vi "Build-timeline.vi"(8 "error in (no error)":errorcluster, 10 "Temp-timeline in":T1={"Previous point"={"Start time [µs]"=0, "End time [µs]"=0, "X [mm]"=0.0, "Y [mm]"=0.0, "Type"=enum."BeginJob", "Speed [mm/µs]"=0.0, "Direction [rad]"=0.0, "X [bit]"=0, "Y [bit]"=0, "Speed [bit/µs]"=0.0, "Power [W]"=0.0, "Power [bit]"=0, "JumpDelay"=0, "MarkDelay"=0, "PolyDelay"=0, "LaserOnDelay"=0, "LaserOffDelay"=0, "LaserPowerDelay"=0, "LaserEnableDelay"=0, "Xraw [mm]"=0.0, "Yraw [mm]"=0.0}, "Current point"={"Start time [µs]"=0, "End time [µs]"=0, "X [mm]"=0.0, "Y [mm]"=0.0, "Type"=enum."BeginJob", "Speed [mm/µs]"=0.0, "Direction [rad]"=0.0, "X [bit]"=0, "Y [bit]"=0, "Speed [bit/µs]"=0.0, "Power [W]"=0.0, "Power [bit]"=0, "JumpDelay"=0, "MarkDelay"=0, "PolyDelay"=0, "LaserOnDelay"=0, "LaserOffDelay"=0, "LaserPowerDelay"=0, "LaserEnableDelay"=0, "Xraw [mm]"=0.0, "Yraw [mm]"=0.0}, "Path"=[], "Current properties"={"ItemID"=0, "Start time"=0, "EffectiveOffset"=[0.0, 0.0], "EffectiveTranfsorm"=[[1.0, 0.0], [0.0, 1.0]], "Z-Offset"=0.0, "Units"=enum."mm", "LaserPower"=0, "Started"=FALSE, "Enabled"=FALSE, "FieldOffset"=[0.0, 0.0], "Offset"=[0.0, 0.0], "TransformEnable"=TRUE, "XYCalFactor"=196.0, "JumpSpeed"={"unit/us"=0.0, "Tick interval us"=0, "Bits per interval"=0}, "MarkSpeed"={"unit/us"=0.0, "Tick interval us"=0, "Bits per interval"=0}}}, 11 "JumpAbs in":refnum<class "JumpRel.lvclass">) -> (0 "error out":errorcluster, 2 "Temp-timeline":T1={"Previous point"={"Start time [µs]"=0, "End time [µs]"=0, "X [mm]"=0.0, "Y [mm]"=0.0, "Type"=enum."BeginJob", "Speed [mm/µs]"=0.0, "Direction [rad]"=0.0, "X [bit]"=0, "Y [bit]"=0, "Speed [bit/µs]"=0.0, "Power [W]"=0.0, "Power [bit]"=0, "JumpDelay"=0, "MarkDelay"=0, "PolyDelay"=0, "LaserOnDelay"=0, "LaserOffDelay"=0, "LaserPowerDelay"=0, "LaserEnableDelay"=0, "Xraw [mm]"=0.0, "Yraw [mm]"=0.0}, "Current point"={"Start time [µs]"=0, "End time [µs]"=0, "X [mm]"=0.0, "Y [mm]"=0.0, "Type"=enum."BeginJob", "Speed [mm/µs]"=0.0, "Direction [rad]"=0.0, "X [bit]"=0, "Y [bit]"=0, "Speed [bit/µs]"=0.0, "Power [W]"=0.0, "Power [bit]"=0, "JumpDelay"=0, "MarkDelay"=0, "PolyDelay"=0, "LaserOnDelay"=0, "LaserOffDelay"=0, "LaserPowerDelay"=0, "LaserEnableDelay"=0, "Xraw [mm]"=0.0, "Yraw [mm]"=0.0}, "Path"=[], "Current properties"={"ItemID"=0, "Start time"=0, "EffectiveOffset"=[0.0, 0.0], "EffectiveTranfsorm"=[[1.0, 0.0], [0.0, 1.0]], "Z-Offset"=0.0, "Units"=enum."mm", "LaserPower"=0, "Started"=FALSE, "Enabled"=FALSE, "FieldOffset"=[0.0, 0.0], "Offset"=[0.0, 0.0], "TransformEnable"=TRUE, "XYCalFactor"=196.0, "JumpSpeed"={"unit/us"=0.0, "Tick interval us"=0, "Bits per interval"=0}, "MarkSpeed"={"unit/us"=0.0, "Tick interval us"=0, "Bits per interval"=0}}}, 3 "JumpAbs out":refnum<class "JumpRel.lvclass">)   [LabVIEW 2013, in "MaterialCharacterization.lvlib" / "JumpRel.lvclass"]
uses:
  JumpRel.lvclass
  ScanParser/Path-buffer.ctl
  ScanParser/Point-buffer.ctl
  Elements.ctl
  ScanParser/Property-buffer.ctl
  ScanParser/Units.ctl
  ScanParser/Speed.ctl
  JumpRel.lvclass/JumpRel.ctl
  <vilib>/Analysis/baseanly.llb/A x Vector.vi
  <vilib>/Analysis/Matrix/Numeric/Conversions/Array To Matrix - RA2.vi
  <vilib>/Analysis/Matrix/NI_Matrix.lvlib
  <vilib>/Analysis/NI_AALBase.lvlib
  Element-XML.lvclass
  ScanParser/MC-ScanParser.lvclass
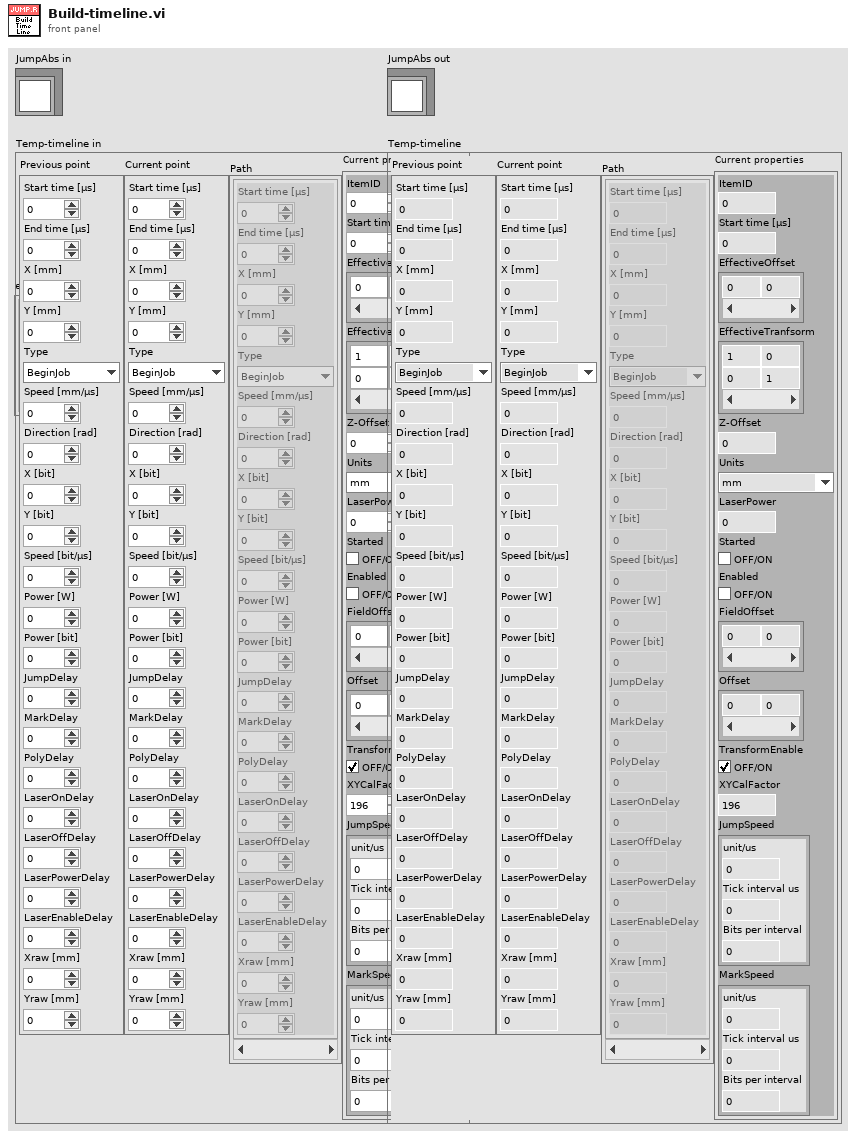
[diagram p1: front panel]
types:
  T1 = typedef "MaterialCharacterization.lvlib/MC-ScanParser.lvclass/Path-buffer.ctl" = cluster{"Previous point":T2, "Current point":T2, "Path":T2[], "Current properties":T4}
  T2 = typedef "MaterialCharacterization.lvlib/MC-ScanParser.lvclass/Point-buffer.ctl" = cluster{"Start time [µs]":i64, "End time [µs]":i64, "X [mm]":dbl, "Y [mm]":dbl, "Type":T3, "Speed [mm/µs]":dbl, "Direction [rad]":dbl, "X [bit]":i16, "Y [bit]":i16, "Speed [bit/µs]":dbl, "Power [W]":dbl, "Power [bit]":u8, "JumpDelay":i64, "MarkDelay":i64, "PolyDelay":i64, "LaserOnDelay":i64, "LaserOffDelay":i64, "LaserPowerDelay":i64, "LaserEnableDelay":i64, "Xraw [mm]":dbl, "Yraw [mm]":dbl}
  T3 = typedef "MaterialCharacterization.lvlib/Element-XML.lvclass/Elements.ctl" = enum16{"BeginJob", "WriteDigital", "WriteAnalog", "Set", "ApplicationEvent", "JumpAbs", "MarkAbs", "JumpRel", "MarkRel", "LongDelay", "EndJob"}
  T4 = typedef "MaterialCharacterization.lvlib/MC-ScanParser.lvclass/Property-buffer.ctl" = cluster{"ItemID":u32, "Start time":i64, "EffectiveOffset":dbl[], "EffectiveTranfsorm":dbl[][], "Z-Offset":sgl, "Units":T5, "LaserPower":u8, "Started":bool, "Enabled":bool, "FieldOffset":dbl[], "Offset":dbl[], "TransformEnable":bool, "XYCalFactor":dbl, "JumpSpeed":T6, "MarkSpeed":T6}
  T5 = typedef "MaterialCharacterization.lvlib/MC-ScanParser.lvclass/Units.ctl" = enum16{"bits", "mm", "inch", "mils"}
  T6 = typedef "MaterialCharacterization.lvlib/MC-ScanParser.lvclass/Speed.ctl" = cluster{"unit/us":dbl, "Tick interval us":u16, "Bits per interval":u16}
  T7 = typedef "NI_Matrix.lvlib/RealMatrix.ctl" = dbl[][]
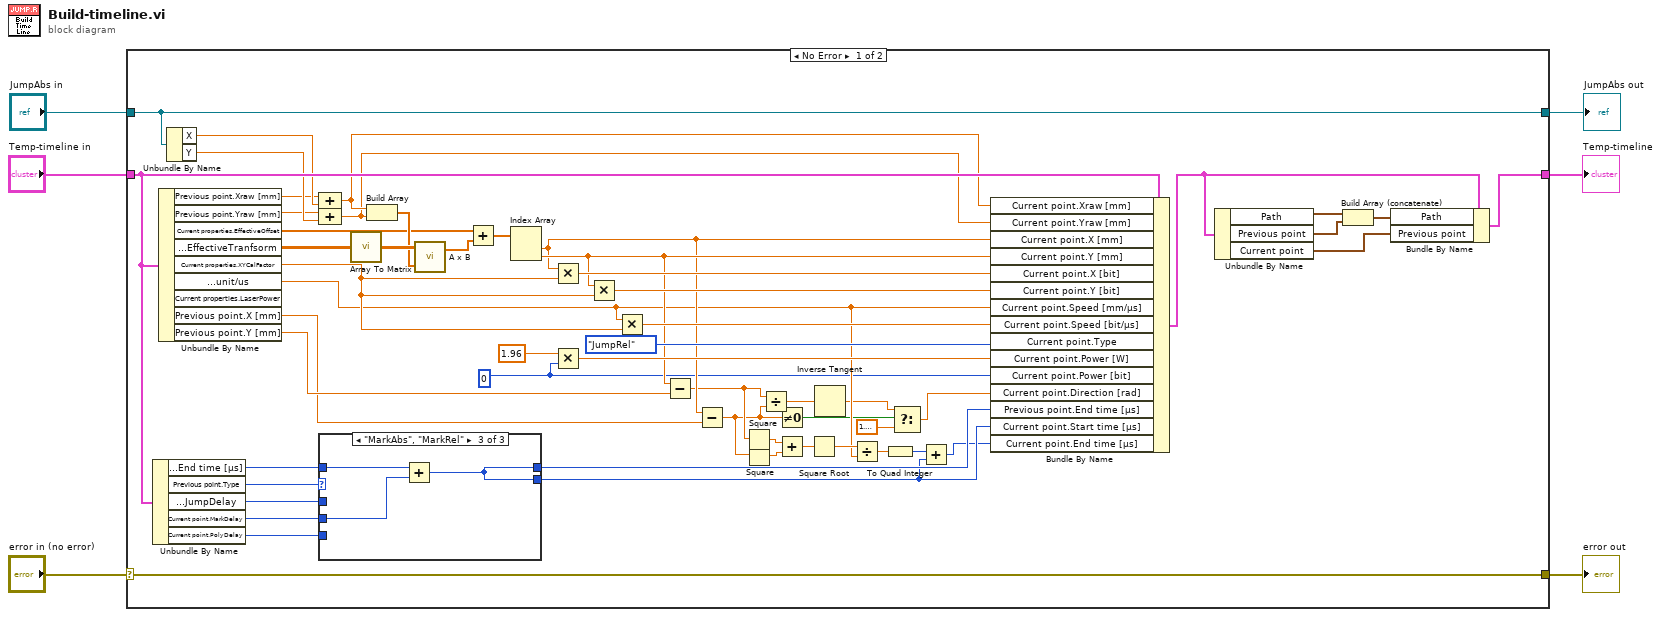
[diagram p0: block diagram]
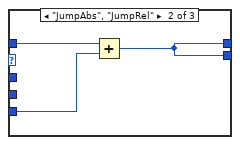
[diagram p3: hidden frame]
diagram:
  n1 = case shown="No Error" "error in (no error)" {
    selector: "error in (no error)" -> [w25 w71]
    tunnel: [w25 w71] -> w5
    tunnel: [w61 w70] -> w3
    tunnel: "JumpAbs in" -> [w61 w70]
    tunnel: "Temp-timeline in" -> [w42 w69]
    tunnel: [w23 w69] -> w1
    frame No Error {
      w18 = u8 0
      n2 = Unbundle By Name(w42) -> ("Previous point.End time [µs]"=w37:i64, "Previous point.Type"=w41:T3, "Current point.JumpDelay"=w40:i64, "Current point.MarkDelay"=w39:i64, "Current point.PolyDelay"=w38:i64)
      n3 = Unbundle By Name(w42) -> ("Previous point.Xraw [mm]"=w15:dbl, "Previous point.Yraw [mm]"=w14:dbl, "Current properties.EffectiveOffset"=w57:dbl[], "Current properties.EffectiveTranfsorm"=w60:dbl[][], "Current properties.XYCalFactor"=w51:dbl, "Current properties.JumpSpeed.unit/us"=w30:dbl, "Previous point.X [mm]"=w44:dbl, "Previous point.Y [mm]"=w46:dbl)  [unwired: 1 out]
      n4 = Unbundle By Name(w61) -> ("X"=w16:dbl, "Y"=w17:dbl)
      n5 = Compound Arithmetic op=ADD(w15, w16) -> (w13:dbl)
      n6 = Compound Arithmetic op=ADD(w14, w17) -> (w12:dbl)
      n7 = case shown="\"MarkAbs\", \"MarkRel\"" w41 {
        tunnel: w40 -> [_ _ _]
        tunnel: w39 -> [_ _ w66]
        tunnel: w38 -> [_ w64 _]
        tunnel: w37 -> [w62 w65 w68]
        tunnel: [w62 w63 w67] -> w36
        tunnel: [w62 w63 w67] -> w27
        frame "BeginJob", Default {
        }
        frame "JumpAbs", "JumpRel" {
          n8 = Add(x=w65, y=w64) -> (x+y=w63:i64)
        }
        frame "MarkAbs", "MarkRel" {
          n9 = Add(x=w68, y=w66) -> (x+y=w67:i64)
        }
      }
      n10 = call-poly <vilib>:"Array To Matrix.vi"("Real 2D Array"=w60) -> ("Real Matrix"=w59:T7)
      n11 = Build Array(w13, w12) -> (w58:dbl[])
      n12 = call-poly <vilib>:"A x B.vi"("Vector"=w58, "A"=w59) -> ("A x Vector"=w56:dbl[])  [unwired: 1 out]
      n13 = Add ("Add.vi")(x=w57, y=w56) -> (x+y=w55:dbl[])
      n14 = Index Array(array=w55) -> (element #1=w45:dbl, element #2=w47:dbl)  [unwired: 2 in]
      n15 = Multiply(x=w45, y=w51) -> (x*y=w54:dbl)
      n16 = Multiply(x=1.96, y=w18) -> (x*y=w49:dbl)
      n17 = Multiply(x=w47, y=w51) -> (x*y=w53:dbl)
      n18 = Multiply(x=w30, y=w51) -> (x*y=w52:dbl)
      n19 = Subtract(x=w47, y=w46) -> (x-y=w32:dbl)
      n20 = Subtract(x=w45, y=w44) -> (x-y=w10:dbl)
      n21 = Square(x=w32) -> (x^2=w35:dbl)
      n22 = Square(x=w10) -> (x^2=w34:dbl)
      n23 = Divide(x=w32, y=w10) -> (x/y=w43:dbl)
      n24 = Not Equal To 0?(x=w10) -> (x != 0?=w9:bool)
      n25 = Add(x=w35, y=w34) -> (x+y=w33:dbl)
      n26 = Square Root(x=w33) -> (sqrt(x)=w31:dbl)
      n27 = Inverse Tangent(1:w43) -> (0:w8:dbl)
      n28 = Divide(x=w31, y=w30) -> (x/y=w29:dbl)
      n29 = To Quad Integer(1:w29) -> (0:w28:i64)
      n30 = Select(t=w8, s=w9, f=1.5707963267948966) -> (s? t:f=w7:dbl)
      n31 = Add(x=w28, y=w27) -> (x+y=w26:i64)
      n32 = Bundle By Name(cluster=w42, "Current point.Xraw [mm]"=w13, "Current point.Yraw [mm]"=w12, "Current point.X [mm]"=w45, "Current point.Y [mm]"=w47, "Current point.X [bit]"=w54, "Current point.Y [bit]"=w53, "Current point.Speed [mm/µs]"=w30, "Current point.Speed [bit/µs]"=w52, "Current point.Type"=Elements."JumpRel", "Current point.Power [W]"=w49, "Current point.Power [bit]"=w18, "Current point.Direction [rad]"=w7, "Previous point.End time [µs]"=w36, "Current point.Start time [µs]"=w27, "Current point.End time [µs]"=w26) -> (w24:T1)
      n33 = Unbundle By Name(w24) -> ("Path"=w22:T2[], "Previous point"=w21:T2, "Current point"=w19:T2)
      n34 = Build Array (concatenate)(w22, w21) -> (w20:T2[])
      n35 = Bundle By Name(cluster=w24, "Path"=w20, "Previous point"=w19) -> (w23:T1)
    }
    frame Error {
    }
  }
  "error out" <- w5
  "JumpAbs out" <- w3
  "Temp-timeline" <- w1
